vi "Set Flowrate.vi"(8 "error in (no error)":errorcluster, 9 "Flowrate, m^3/s":dbl, 11 "Pump in":T1) -> (0 "error out":errorcluster, 3 "Pump out":T1)   [LabVIEW 2017, in "Pump Controller.lvlib"]
uses:
  Pump Controller.lvlib
  Controls/Pump.ctl
  <instrlib>/Roboteq Controller KBL1xxx/Public/Controls/Controller.ctl
  <instrlib>/Roboteq Controller KBL1xxx/Roboteq Controller KBL1xxx.lvlib
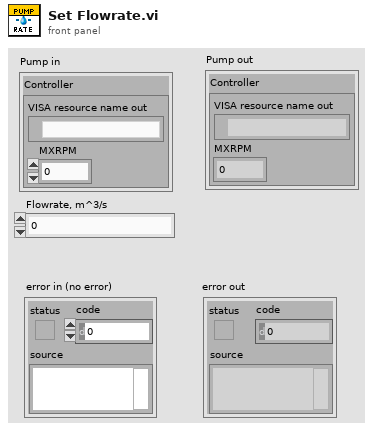
[diagram p1: front panel]
types:
  T1 = typedef "Pump Controller.lvlib/Pump.ctl" = cluster{"Controller":T2}
  T2 = typedef "Roboteq Controller KBL1xxx.lvlib/Controller.ctl" = cluster{"VISA resource name out":refnum<visa-resource-name>, "MXRPM":u16}
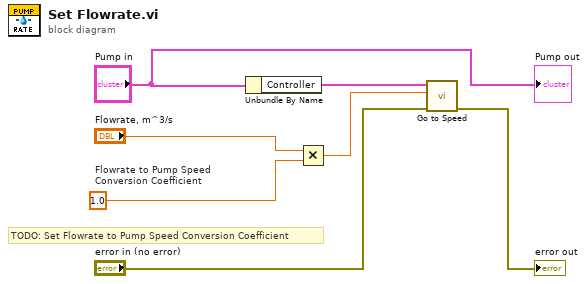
[diagram p0: block diagram]
diagram:
  w6 = 1.0  # Flowrate to Pump Speed Conversion Coefficient
  # "TODO: Set Flowrate to Pump Speed Conversion Coefficient"
  n1 = Unbundle By Name("Pump in") -> ("Controller"=w5:T2)
  n2 = Multiply(x="Flowrate, m^3/s", y=w6) -> (x*y=w4:dbl)
  n3 = call <instrlib>:"Go to Speed.vi"("error in (no error)"="error in (no error)", "Speed, RPM"=w4, "Controller in"=w5) -> ("error out"=→"error out":errorcluster)  [unwired: 6 in, 2 out]
  "Pump out" <- "Pump in"
